vi "rszvl_core_global.vi"() -> ()   [LabVIEW 2014] (continued)
the settings of Bluetooth measurements.\n\n(2) Results (Class):\nAttributes that return the measured values and measurement results.", "Flags"={"OPC Wait"=FALSE, "Dont check status"=FALSE, "*WAI"=FALSE}, "Check Status Callback"=""}, {"Level"=2, "Descriptive Name"="Settings", "Class Only"=TRUE, "Data Type"=0, "Access"=0, "Identifier"="", "Range Table"="", "Command"="", "Read Callback"="", "Write Callback"="", "Range Callback"="", "Check Callback"="", "Rngtable Callback"="", "Coerce Callback"="", "User Callback"="", "Supported Models"="", "Instrument Options"="", "Repeated Capabilities"="", "Restricted Repeated Capabilities"="", "Help"="Attributes that configure the settings of Bluetooth measurements.\n\n(1) BTO Packet Type:\nThis attribute selects the packet type to be measured.\n\n(2) BTO Samples Per Symbols:\nThis attribute selects the number of measurement samples (points) per symbol for the measurement.\n\n(3) BTO Output Power Class:\nThis attribute selects the power class for the Output Power measurement. The power class defines the limits for the Output Power measurement.\n\n(4) BTO Position of Average Power:\nThis attribute defines the start/stop position for the calculation of the average power of a burst.\n\n(5) BTO Resolution Bandwidth Auto:\nThis attribute links the resolution bandwidth to the settings according to the RF Test Specification.\n\n(6) BTO Resolution Bandwidth:\nThis attribute sets the resolution bandwidth of the analyzer for the currently selected Bluetooth\nmeasurement\n\n(7) BTO Video Bandwidth Auto:\nThis attribute links the video bandwidth to the settings according to the RF Test Specification.\n\n(8) BTO Video Bandwidth:\nThis attribute sets the video bandwidth for the currently selected Bluetooth measurement.\n\n(9) BTO Measurement Filter:\nThis attribute selects the receive filter for the signal to measure.\n\n(10) BTO Trace Mode:\nThis attribute defines the way of displaying and evaluating the measurement curves for the\nselected Bluetooth measurement.\n\n(11) BTO Select Trace:\nThis attribute selects the measurement curve for evaluation of the modulation characteristics.\n\n(12) BTO Trace Detector:\nThis attribute selects the detector for the currently selected Bluetooth measurement. The numeric suffix assigns the detector to a trace.\n\n(13) BTO Sweep Count:\nThis attribute defines the number of sweeps for the currently selected Bluetooth measurement.\nThis number will be started as a single sweep.\n\n(14) BTO Sweep Time Auto:\nThis attribute links the sweep time to the settings according to the RF Test Specification.\n\n(15) BTO Sweep Time:\nThis attribute defines the duration of a sweep sequence for the active Bluetooth measurement.\n\n(16) BTO Mode:\nThis attribute selects the Bluetooth analyzer mode.\n\n(17) BTO Measurement Mode:\nThis attribute selects the current measurement according to the Bluetooth standard.\n\n(18) BTO Lowest 24 Bits of Bluetooth Device Address:\nThis attribute sets the lowest 24 bits of Bluetooth Device Address. These bits are used to determine the begin of the signal packet.\n\n(19) BTO Frequency Channel:\nThis attribute selects the frequency channel for the measurements according to the Bluetooth standard.\n\nNote:\nRange Tables rszvl_rngBtoChannel and rszvl_rngBtoChannelFranc are used for range checking.\n\n(20) BTO Number of Adjacent Channels:\nThis attribute selects the number of adjacent channel pairs during the measurement of the\nadjacent channel power. The number of adjacent channels will be limited as soon as the border of\nthe Bluetooth frequency band is reached.\n\n(21) BTO Geographical Region:\nThis attribute selects the geographical region for the measurements. The region determines the number of available frequency channels.\n\n(22) BTO Antenna Gain:\nThis attribute defines an external gain known to the analyzer, which will take it into account during\nthe display of measurement results. With this function the gain of an antenna or of an external\npreamplifier can be taken into account for the measurement values.\n\n(23) BTO Burst Offset:\nThis attribute defines the time to be recorded before a signal burst is recognized.\n\n(24) BTO Find Burst State:\nThis attribute switches the search for a signal burst on or off.\n\n(25) BTO Sync Offset:\nThis attribute defines the number of bits to be recorded before the first preamble bit is detected.\n\n(26) BTO Find Sync State:\nThis attribute switches the search for a sync pattern on or off.\n\n(27) BTO Search Time:\nThis attribute selects manual setting of the record length and defines the record length to be used\nfor the search of sync word and burst. The input of the record length is expected in seconds.\n\n(28) BTO Search Time Auto:\nThis attribute activates the automatic setting of the record length for the sync word and burst\nsearch, depending on the selected packet type.\n\n(29) BTO Carrier Frequency Stability Block Count:\nThis attribute sets the number of blocks to be measured.\n\nNote: \n\n(1) This command is only available with active Carrier Frequency Stability and Modulation Accuracy measurement\n\n(30) BTO Spurious Emissions Adjacent Channels:\nThis attribute selects the number of adjacent channel pairs during the In–band Spurious Emissions measurement. The number of adjacent channels will be limited as soon as the border of the Bluetooth frequency band is reached.\n\nNote: \n\n(1) This command is only available with active In–band Spurious Emissions measurement\n\n(31) BTO Spurious Emissions Gate Auto:\nThis attribute adjusts the gate settings for the In–band Spurious Emissions automatically.\n\nNote:\n\n(1) This command is only available with active In–band Spurious Emissions measurement\n\n(32) BTO Packet Bytes SCO:\nThis attribute selects the number of payload bytes that are transmitted in a packet.\n\n(33) BTO Relative Transimt Power Time:\nThis attribute sets the start/stop time for the power measurement of the DPSK or GFSK sections of the packet.\n\nNote: \n\n(1) This command is only available with active Relative Transmit Power measurement\n\n(34) BTO Y axis Scaling:\nThis attribute defines the scaling of the y–axis in the currently selected unit.\n\n(35) BTO Zoom:\nThis attribute enables or disables the zoom function.\n\nNote: \n\n(1) The zoom function is only available for the Output Power, Modulation Characteristics, Initial Carrier Frequency Tolerance, and Carrier Frequency Drift measurements.\n\n(36) BTO Zoom Start:\nThis attribute sets the start time for the display of individual measured values.\n\nNote: \n\n(1) The zoom function is only available for the Output Power, Modulation Characteristics, Initial Carrier Frequency Tolerance, and Carrier Frequency Drift measurements.", "Flags"={"OPC Wait"=FALSE, "Dont check status"=FALSE, "*WAI"=FALSE}, "Check Status Callback"=""}, {"Level"=3, "Descriptive Name"="BTO Packet Type", "Class Only"=FALSE, "Data Type"=0, "Access"=2, "Identifier"="RSZVL_ATTR_BTO_PTYPE", "Range Table"="rszvl_rngBtoWritePtype", "Command"="CONF:BTO:PTYP", "Read Callback"="", "Write Callback"="", "Range Callback"="", "Check Callback"="", "Rngtable Callback"="", "Coerce Callback"="", "User Callback"="", "Supported Models"="", "Instrument Options"="", "Repeated Capabilities"="", "Restricted Repeated Capabilities"="", "Help"="This attribute selects the packet type to be measured.\n\nAvailable Repeated Capabilities:\nNone\n\nRemote-control command(s):\nCONFigure:BTOoth:PTYPe DH1 | DH3 | DH5 | AUTO", "Flags"={"OPC Wait"=FALSE, "Dont check status"=FALSE, "*WAI"=FALSE}, "Check Status Callback"=""}, {"Level"=3, "Descriptive Name"="BTO Samples Per Symbols", "Class Only"=FALSE, "Data Type"=0, "Access"=2, "Identifier"="RSZVL_ATTR_BTO_PRAT", "Range Table"="rszvl_rngBtoPrat", "Command"="CONF:BTO:PRAT", "Read Callback"="", "Write Callback"="", "Range Callback"="", "Check Callback"="", "Rngtable Callback"="", "Coerce Callback"="", "User Callback"="", "Supported Models"="", "Instrument Options"="", "Repeated Capabilities"="", "Restricted Repeated Capabilities"="", "Help"="This attribute selects the number of measurement samples (points) per symbol for the measurement.\n\nAvailable Repeated Capabilities:\nNone\n\nRemote-control command(s):\nCONFigure:BTOoth:PRATe", "Flags"={"OPC Wait"=FALSE, "Dont check status"=FALSE, "*WAI"=FALSE}, "Check Status Callback"=""}, {"Level"=3, "Descriptive Name"="BTO Output Power Class", "Class Only"=FALSE, "Data Type"=0, "Access"=2, "Identifier"="RSZVL_ATTR_BTO_PCL", "Range Table"="rszvl_rngBtoPcl", "Command"="CONF:BTO:PCL", "Read Callback"="", "Write Callback"="", "Range Callback"="", "Check Callback"="", "Rngtable Callback"="", "Coerce Callback"="", "User Callback"="", "Supported Models"="", "Instrument Options"="", "Repeated Capabilities"="", "Restricted Repeated Capabilities"="", "Help"="This attribute selects the power class for the Output Power measurement. The power class defines the limits for the Output Power measurement.\n\nAvailable Repeated Capabilities:\nNone\n\nRemote-control command(s):\nCONFigure:BTOoth:PCLass", "Flags"={"OPC Wait"=FALSE, "Dont check status"=FALSE, "*WAI"=FALSE}, "Check Status Callback"=""}, {"Level"=3, "Descriptive Name"="BTO Position of Average Power", "Class Only"=FALSE, "Data Type"=1, "Access"=2, "Identifier"="RSZVL_ATTR_BTO_POW_AVER", "Range Table"="rszvl_rngPct", "Command"="CONF:BTO:POW:AVER:{ModifStopStart}", "Read Callback"="", "Write Callback"="", "Range Callback"="", "Check Callback"="", "Rngtable Callback"="", "Coerce Callback"="", "User Callback"="", "Supported Models"="", "Instrument Options"="", "Repeated Capabilities"="", "Restricted Repeated Capabilities"="", "Help"="This attribute defines the start/stop position for the calculation of the average power of a burst.\n\nAvailable Repeated Capabilities:\nModifStopStart: Stop,Start\r\n\nRemote-control command(s):\nCONFigure:BTOoth:POWer:AVERage:STARt|STOP", "Flags"={"OPC Wait"=FALSE, "Dont check status"=FALSE, "*WAI"=FALSE}, "Check Status Callback"=""}, {"Level"=3, "Descriptive Name"="BTO Resolution Bandwidth Auto", "Class Only"=FALSE, "Data Type"=3, "Access"=2, "Identifier"="RSZVL_ATTR_BTO_BWID_AUTO", "Range Table"="", "Command"="CONF:BTO:BWID:AUTO", "Read Callback"="", "Write Callback"="", "Range Callback"="", "Check Callback"="", "Rngtable Callback"="", "Coerce Callback"="", "User Callback"="", "Supported Models"="", "Instrument Options"="", "Repeated Capabilities"="", "Restricted Repeated Capabilities"="", "Help"="This attribute links the resolution bandwidth to the settings according to the RF Test Specification.\n\nAvailable Repeated Capabilities:\nNone\n\nRemote-control command(s):\nCONFigure:BTOoth:BANDwidth|BWIDth[:RESolution]:AUTO ON | OFF", "Flags"={"OPC Wait"=TRUE, "Dont check status"=FALSE, "*WAI"=FALSE}, "Check Status Callback"=""}, {"Level"=3, "Descriptive Name"="BTO Resolution Bandwidth", "Class Only"=FALSE, "Data Type"=1, "Access"=2, "Identifier"="RSZVL_ATTR_BTO_BWID", "Range Table"="rszvl_rngBtoBwid", "Command"="CONF:BTO:BWID:RES", "Read Callback"="", "Write Callback"="", "Range Callback"="", "Check Callback"="", "Rngtable Callback"="", "Coerce Callback"="", "User Callback"="", "Supported Models"="", "Instrument Options"="", "Repeated Capabilities"="", "Restricted Repeated Capabilities"="", "Help"="This attribute sets the resolution bandwidth of the analyzer for the currently selected Bluetooth\nmeasurement\n\nAvailable Repeated Capabilities:\nNone\n\nRemote-control command(s):\nCONFigure:BTOoth:BANDwidth|BWIDth[:RESolution]", "Flags"={"OPC Wait"=FALSE, "Dont check status"=FALSE, "*WAI"=FALSE}, "Check Status Callback"=""}, {"Level"=3, "Descriptive Name"="BTO Video Bandwidth Auto", "Class Only"=FALSE, "Data Type"=3, "Access"=2, "Identifier"="RSZVL_ATTR_BTO_VID_AUTO", "Range Table"="", "Command"="CONF:BTO:BWID:VID:AUTO", "Read Callback"="", "Write Callback"="", "Range Callback"="", "Check Callback"="", "Rngtable Callback"="", "Coerce Callback"="", "User Callback"="", "Supported Models"="", "Instrument Options"="", "Repeated Capabilities"="", "Restricted Repeated Capabilities"="", "Help"="This attribute links the video bandwidth to the settings according to the RF Test Specification.\n\nAvailable Repeated Capabilities:\nNone\n\nRemote-control command(s):\nCONFigure:BTOoth:BANDwidth|BWIDth:VIDeo:AUTO ON | OFF", "Flags"={"OPC Wait"=TRUE, "Dont check status"=FALSE, "*WAI"=FALSE}, "Check Status Callback"=""}, {"Level"=3, "Descriptive Name"="BTO Video Bandwidth", "Class Only"=FALSE, "Data Type"=1, "Access"=2, "Identifier"="RSZVL_ATTR_BTO_VID", "Range Table"="rszvl_rngBtoVideo", "Command"="CONF:BTO:BWID:VID", "Read Callback"="", "Write Callback"="", "Range Callback"="", "Check Callback"="", "Rngtable Callback"="", "Coerce Callback"="", "User Callback"="", "Supported Models"="", "Instrument Options"="", "Repeated Capabilities"="", "Restricted Repeated Capabilities"="", "Help"="This attribute sets the video bandwidth for the currently selected Bluetooth measurement.\n\nAvailable Repeated Capabilities:\nNone\n\nRemote-control command(s):\nCONFigure:BTOoth:BANDwidth|BWIDth:VIDeo", "Flags"={"OPC Wait"=FALSE, "Dont check status"=FALSE, "*WAI"=FALSE}, "Check Status Callback"=""}, {"Level"=3, "Descriptive Name"="BTO Measurement Filter", "Class Only"=FALSE, "Data Type"=0, "Access"=2, "Identifier"="RSZVL_ATTR_BTO_FILT_MEAS", "Range Table"="rszvl_rngBtoMeasFilt", "Command"="DDEM:FILT:MEAS", "Read Callback"="", "Write Callback"="", "Range Callback"="", "Check Callback"="", "Rngtable Callback"="", "Coerce Callback"="", "User Callback"="", "Supported Models"="", "Instrument Options"="", "Repeated Capabilities"="", "Restricted Repeated Capabilities"="", "Help"="This attribute selects the receive filter for the signal to measure.\n\nAvailable Repeated Capabilities:\nNone\n\nRemote-control command(s):\n[SENSe<1|2>:]DDEMod:FILTer:MEASurement OFF | BTOoth", "Flags"={"OPC Wait"=FALSE, "Dont check status"=FALSE, "*WAI"=FALSE}, "Check Status Callback"=""}, {"Level"=3, "Descriptive Name"="BTO Trace Mode", "Class Only"=FALSE, "Data Type"=0, "Access"=2, "Identifier"="RSZVL_ATTR_BTO_TRAC_MOD", "Range Table"="rszvl_rngTraceModeWithBlank", "Command"="CONF:BTO:TRAC{Trace}:MODE", "Read Callback"="", "Write Callback"="", "Range Callback"="", "Check Callback"="", "Rngtable Callback"="", "Coerce Callback"="", "User Callback"="", "Supported Models"="", "Instrument Options"="", "Repeated Capabilities"="", "Restricted Repeated Capabilities"="", "Help"="This attribute defines the way of displaying and evaluating the measurement curves for the selected Bluetooth measurement.\n\nAvailable Repeated Capabilities:\nTrace: TR1,TR2,TR3,TR4,TR5,TR6,TR7,TR8,TR9,TR10,TR11,TR12,TR13,TR14,TR15,TR16,TR17,TR18,TR19,TR20\r\n\nRemote-control command(s):\nCONFigure:BTOoth:TRACe<1...3>:MODE WRITe | VIEW | AVERage | BLANk | MAXHold | MINHold", "Flags"={"OPC Wait"=FALSE, "Dont check status"=FALSE, "*WAI"=FALSE}, "Check Status Callback"=""}, {"Level"=3, "Descriptive Name"="BTO Select Trace", "Class Only"=FALSE, "Data Type"=4, "Access"=1, "Identifier"="RSZVL_ATTR_BTO_TRAC", "Range Table"="", "Command"="CONF:BTO:TRAC{Trace}:SEL", "Read Callback"="", "Write Callback"="", "Range Callback"="", "Check Callback"="", "Rngtable Callback"="", "Coerce Callback"="", "User Callback"="", "Supported Models"="", "Instrument Options"="", "Repeated Capabilities"="", "Restricted Repeated Capabilities"="", "Help"="This attribute selects the measurement curve for evaluation of the modulation characteristics.\n\nAvailable Repeated Capabilities:\nTrace: TR1,TR2,TR3,TR4,TR5,TR6,TR7,TR8,TR9,TR10,TR11,TR12,TR13,TR14,TR15,TR16,TR17,TR18,TR19,TR20\r\n\nRemote-control command(s):\nCONFigure:BTOoth:TRACe<1...6>:SELect", "Flags"={"OPC Wait"=FALSE, "Dont check status"=FALSE, "*WAI"=FALSE}, "Check Status Callback"=""}, {"Level"=3, "Descriptive Name"="BTO Trace Detector", "Class Only"=FALSE, "Data Type"=0, "Access"=2, "Identifier"="RSZVL_ATTR_BTO_TRAC_DET", "Range Table"="rszvl_rngBtoTraceDetector", "Command"="CONF:BTO:DET{Trace}", "Read Callback"="", "Write Callback"="", "Range Callback"="", "Check Callback"="", "Rngtable Callback"="", "Coerce Callback"="", "User Callback"="", "Supported Models"="", "Instrument Options"="", "Repeated Capabilities"="", "Restricted Repeated Capabilities"="", "Help"="This attribute selects the detector for the currently selected Bluetooth measurement. The numeric suffix assigns the detector to a trace.\n\nAvailable Repeated Capabilities:\nTrace: TR1,TR2,TR3,TR4,TR5,TR6,TR7,TR8,TR9,TR10,TR11,TR12,TR13,TR14,TR15,TR16,TR17,TR18,TR19,TR20\r\n\nRemote-control command(s):\nCONFigure:BTOoth:DETector<1...4> APEak | NEGative | POSitive |SAMPle | RMS | AVERage", "Flags"={"OPC Wait"=FALSE, "Dont check status"=FALSE, "*WAI"=FALSE}, "Check Status Callback"=""}, {"Level"=3, "Descriptive Name"="BTO Sweep Count", "Class Only"=FALSE, "Data Type"=0, "Access"=2, "Identifier"="RSZVL_ATTR_BTO_SWE", "Range Table"="rszvl_rngSweepCount", "Command"="CONF:BTO:SWE:COUN", "Read Callback"="", "Write Callback"="", "Range Callback"="", "Check Callback"="", "Rngtable Callback"="", "Coerce Callback"="", "User Callback"="", "Supported Models"="", "Instrument Options"="", "Repeated Capabilities"="", "Restricted Repeated Capabilities"="", "Help"="This attribute defines the number of sweeps for the currently selected Bluetooth measurement.\nThis number will be started as a single sweep.\n\nAvailable Repeated Capabilities:\nNone\n\nRemote-control command(s):\nCONFigure:BTOoth:SWEep:COUNt", "Flags"={"OPC Wait"=FALSE, "Dont check status"=FALSE, "*WAI"=FALSE}, "Check Status Callback"=""}, {"Level"=3, "Descriptive Name"="BTO Sweep Time Auto", "Class Only"=FALSE, "Data Type"=3, "Access"=2, "Identifier"="RSZVL_ATTR_BTO_SWE_TIME_AUTO", "Range Table"="", "Command"="CONF:BTO:SWE:TIME:AUTO", "Read Callback"="", "Write Callback"="", "Range Callback"="", "Check Callback"="", "Rngtable Callback"="", "Coerce Callback"="", "User Callback"="", "Supported Models"="", "Instrument Options"="", "Repeated Capabilities"="", "Restricted Repeated Capabilities"="", "Help"="This attribute links the sweep time to the settings according to the RF Test Specification.\n\nAvailable Repeated Capabilities:\nNone\n\nRemote-control command(s):\nCONFigure:BTOoth:SWEep:TIME:AUTO ON | OFF", "Flags"={"OPC Wait"=TRUE, "Dont check status"=FALSE, "*WAI"=FALSE}, "Check Status Callback"=""}, {"Level"=3, "Descriptive Name"="BTO Sweep Time", "Class Only"=FALSE, "Data Type"=1, "Access"=2, "Identifier"="RSZVL_ATTR_BTO_SWE_TIME", "Range Table"="", "Command"="CONF:BTO:SWE:TIME", "Read Callback"="", "Write Callback"="", "Range Callback"="", "Check Callback"="", "Rngtable Callback"="", "Coerce Callback"="", "User Callback"="", "Supported Models"="", "Instrument Options"="", "Repeated Capabilities"="", "Restricted Repeated Capabilities"="", "Help"="This attribute defines the duration of a sweep sequence for the active Bluetooth measurement.\n\nAvailable Repeated Capabilities:\nNone\n\nRemote-control command(s):\nCONFigure:BTOoth:SWEep:TIME", "Flags"={"OPC Wait"=FALSE, "Dont check status"=FALSE, "*WAI"=FALSE}, "Check Status Callback"=""}, {"Level"=3, "Descriptive Name"="BTO Mode", "Class Only"=FALSE, "Data Type"=4, "Access"=1, "Identifier"="RSZVL_ATTR_BTO_MODE", "Range Table"="", "Command"="INST:SEL BTO", "Read Callback"="", "Write Callback"="", "Range Callback"="", "Check Callback"="", "Rngtable Callback"="", "Coerce Callback"="", "User Callback"="", "Supported Models"="", "Instrument Options"="", "Repeated Capabilities"="", "Restricted Repeated Capabilities"="", "Help"="This attribute selects the Bluetooth analyzer mode.\n\nAvailable Repeated Capabilities:\nNone\n\nRemote-control command(s):\nINSTrument<1|2>:SELect BTOoth", "Flags"={"OPC Wait"=FALSE, "Dont check status"=FALSE, "*WAI"=FALSE}, "Check Status Callback"=""}, {"Level"=3, "Descriptive Name"="BTO Measurement Mode", "Class Only"=FALSE, "Data Type"=0, "Access"=2, "Identifier"="RSZVL_ATTR_BTO", "Range Table"="rszvl_rngBtoMeasMode", "Command"="CONF:BTO:MEAS", "Read Callback"="", "Write Callback"="", "Range Callback"="", "Check Callback"="", "Rngtable Callback"="", "Coerce Callback"="", "User Callback"="", "Supported Models"="", "Instrument Options"="", "Repeated Capabilities"="", "Restricted Repeated Capabilities"="", "Help"="This attribute selects the current measurement according to the Bluetooth standard.\n\nAvailable Repeated Capabilities:\nNone\n\nRemote-control command(s):\nCONFigure:BTOoth:MEASurement OPOWer | ACLR | MCHar | ICFTolerance | CFDRift | RTPower | IBSemissions | DPENcoding | CFSTability", "Flags"={"OPC Wait"=FALSE, "Dont check status"=FALSE, "*WAI"=FALSE}, "Check Status Callback"=""}, {"Level"=3, "Descriptive Name"="BTO Lowest 24 Bits of Bluetooth Device Address", "Class Only"=FALSE, "Data Type"=0, "Access"=2, "Identifier"="RSZVL_ATTR_BTO_LAP", "Range Table"="", "Command"="SENS1:DDEM:SEAR:SYNC:LAP", "Read Callback"="rszvl_hex_ReadCallback.vi", "Write Callback"="rszvl_hex_WriteCallback.vi", "Range Callback"="", "Check Callback"="", "Rngtable Callback"="", "Coerce Callback"="", "User Callback"="", "Supported Models"="", "Instrument Options"="", "Repeated Capabilities"="", "Restricted Repeated Capabilities"="", "Help"="This attribute sets the lowest 24 bits of Bluetooth Device Address. These bits are used to determine the begin of the signal packet.\n\nAvailable Repeated Capabilities:\nNone\n\nRemote-control command(s):\n[SENSe<1|2>:]DDEMod:SEARch:SYNC:LAP", "Flags"={"OPC Wait"=FALSE, "Dont check status"=FALSE, "*WAI"=FALSE}, "Check Status Callback"=""}, {"Level"=3, "Descriptive Name"="BTO Frequency Channel", "Class Only"=FALSE, "Data Type"=0, "Access"=2, "Identifier"="RSZVL_ATTR_BTO_CHANNEL", "Range Table"="rszvl_rngBtoChannel", "Command"="CONF:BTO:CHAN", "Read Callback"="", "Write Callback"="", "Range Callback"="", "Check Callback"="", "Rngtable Callback"="", "Coerce Callback"="", "User Callback"="", "Supported Models"="", "Instrument Options"="", "Repeated Capabilities"="", "Restricted Repeated Capabilities"="", "Help"="This attribute selects the frequency channel for the measurements according to the Bluetooth standard.\n\nAvailable Repeated Capabilities:\nNone\n\nRemote-control command(s):\nCONFigure:BTOoth:CHANnel", "Flags"={"OPC Wait"=FALSE, "Dont check status"=FALSE, "*WAI"=FALSE}, "Check Status Callback"=""}, {"Level"=3, "Descriptive Name"="BTO Number of Adjacent Channels", "Class Only"=FALSE, "Data Type"=0, "Access"=2, "Identifier"="RSZVL_ATTR_BTO_ACLR_ACP", "Range Table"="rszvl_rngBtoAclrAcp", "Command"="CONF:BTO:ACLR:ACP", "Read Callback"="", "Write Callback"="", "Range Callback"="", "Check Callback"="", "Rngtable Callback"="", "Coerce Callback"="", "User Callback"="", "Supported Models"="", "Instrument Options"="", "Repeated Capabilities"="", "Restricted Repeated Capabilities"="", "Help"="This attribute selects the number of adjacent channel pairs during the measurement of the\nadjacent channel power. The number of adjacent channels will be limited as soon as the border of\nthe Bluetooth frequency band is reached.\n\nAvailable Repeated Capabilities:\nNone\n\nRemote-control command(s):\nCONFigure:BTOoth:ACLR:ACPairs", "Flags"={"OPC Wait"=FALSE, "Dont check status"=FALSE, "*WAI"=FALSE}, "Check Status Callback"=""}, {"Level"=3, "Descriptive Name"="BTO Antenna Gain", "Class Only"=FALSE, "Data Type"=1, "Access"=2, "Identifier"="RSZVL_ATTR_BTO_EGA_INP", "Range Table"="rszvl_rngBtoAntennaGain", "Command"="CORR:EGA:INP", "Read Callback"="", "Write Callback"="", "Range Callback"="", "Check Callback"="", "Rngtable Callback"="", "Coerce Callback"="", "User Callback"="", "Supported Models"="", "Instrument Options"="", "Repeated Capabilities"="", "Restricted Repeated Capabilities"="", "Help"="This attribute defines an external gain known to the analyzer, which will take it into account during\nthe display of measurement results. With this function the gain of an antenna or of an external\npreamplifier can be taken into account for the measurement values.\n\nAvailable Repeated Capabilities:\nNone\n\nRemote-control command(s):\n[SENSe<1|2>:]CORRection:EGAin:INPut[:MAGNitude]", "Flags"={"OPC Wait"=FALSE, "Dont check status"=FALSE, "*WAI"=FALSE}, "Check Status Callback"=""}, {"Level"=3, "Descriptive Name"="BTO Burst Offset", "Class Only"=FALSE, "Data Type"=1, "Access"=2, "Identifier"="RSZVL_ATTR_BTO_PULS_OFFS", "Range Table"="rszvl_rngBtoBurstOffs", "Command"="DDEM:SEAR:PULS:OFFS", "Read Callback"="", "Write Callback"="", "Range Callback"="", "Check Callback"="", "Rngtable Callback"="", "Coerce Callback"="", "User Callback"="", "Supported Models"="", "Instrument Options"="", "Repeated Capabilities"="", "Restricted Repeated Capabilities"="", "Help"="This attribute defines the time to be recorded before a signal burst is recognized.\n\nAvailable Repeated Capabilities:\nNone\n\nRemote-control command(s):\n[SENSe<1|2>:]DDEMod:SEARch:PULSe:OFFSet", "Flags"={"OPC Wait"=FALSE, "Dont check status"=FALSE, "*WAI"=FALSE}, "Check Status Callback"=""}, {"Level"=3, "Descriptive Name"="BTO Find Burst State", "Class Only"=FALSE, "Data Type"=3, "Access"=2, "Identifier"="RSZVL_ATTR_BTO_SEARCH_PULS", "Range Table"="", "Command"="DDEM:SEAR:PULS", "Read Callback"="", "Write Callback"="", "Range Callback"="", "Check Callback"="", "Rngtable Callback"="", "Coerce Callback"="", "User Callback"="", "Supported Models"="", "Instrument Options"="", "Repeated Capabilities"="", "Restricted Repeated Capabilities"="", "Help"="This attribute switches the search for a signal burst on or off.\n\nAvailable Repeated Capabilities:\nNone\n\nRemote-control command(s):\n[SENSe<1|2>:]DDEMod:SEARch:PULSe[:STATe] ON | OFF", "Flags"={"OPC Wait"=FALSE, "Dont check status"=FALSE, "*WAI"=FALSE}, "Check Status Callback"=""}, {"Level"=3, "Descriptive Name"="BTO Sync Offset", "Class Only"=FALSE, "Data Type"=0, "Access"=2, "Identifier"="RSZVL_ATTR_BTO_SYNC_OFFS", "Range Table"="rszvl_rngBtoSyncOffs", "Command"="DDEM:SEAR:SYNC:OFFS", "Read Callback"="", "Write Callback"="", "Range Callback"="", "Check Callback"="", "Rngtable Callback"="", "Coerce Callback"="", "User Callback"="", "Supported Models"="", "Instrument Options"="", "Repeated Capabilities"="", "Restricted Repeated Capabilities"="", "Help"="This attribute defines the number of bits to be recorded before the first preamble bit is detected.\n\nAvailable Repeated Capabilities:\nNone\n\nRemote-control command(s):\n[SENSe<1|2>:]DDEMod:SEARch:SYNC:OFFSet", "Flags"={"OPC Wait"=FALSE, "Dont check status"=FALSE, "*WAI"=FALSE}, "Check Status Callback"=""}, {"Level"=3, "Descriptive Name"="BTO Find Sync State", "Class Only"=FALSE, "Data Type"=3, "Access"=2, "Identifier"="RSZVL_ATTR_BTO_SEARCH_SYNC", "Range Table"="", "Command"="DDEM:SEAR:SYNC", "Read Callback"="", "Write Callback"="", "Range Callback"="", "Check Callback"="", "Rngtable Callback"="", "Coerce Callback"="", "User Callback"="", "Supported Models"="", "Instrument Options"="", "Repeated Capabilities"="", "Restricted Repeated Capabilities"="", "Help"="This attribute switches the search for a sync pattern on or off.\n\nAvailable Repeated Capabilities:\nNone\n\nRemote-control command(s):\n[SENSe<1|2>:]DDEMod:SEARch:SYNC[:STATe]", "Flags"={"OPC Wait"=FALSE, "Dont check status"=FALSE, "*WAI"=FALSE}, "Check Status Callback"=""}, {"Level"=3, "Descriptive Name"="BTO Search Time", "Class Only"=FALSE, "Data Type"=1, "Access"=2, "Identifier"="RSZVL_ATTR_BTO_SEARCH_TIME", "Range Table"="rszvl_rngBtoSearchTime", "Command"="DDEM:SEAR:TIME", "Read Callback"="", "Write Callback"="", "Range Callback"="", "Check Callback"="", "Rngtable Callback"="", "Coerce Callback"="", "User Callback"="", "Supported Models"="", "Instrument Options"="", "Repeated Capabilities"="", "Restricted Repeated Capabilities"="", "Help"="This attribute selects manual setting of the record length and defines the record length to be used\nfor the search of sync word and burst. The input of the record length is expected in seconds.\n\nAvailable Repeated Capabilities:\nNone\n\nRemote-control command(s):\n[SENSe<1|2>:]DDEMod:SEARch:TIME", "Flags"={"OPC Wait"=FALSE, "Dont check status"=FALSE, "*WAI"=FALSE}, "Check Status Callback"=""}, {"Level"=3, "Descriptive Name"="BTO Search Time Auto", "Class Only"=FALSE, "Data Type"=3, "Access"=2, "Identifier"="RSZVL_ATTR_BTO_SEARCH_TIME_AUTO", "Range Table"="", "Command"="DDEM:SEAR:TIME:AUTO", "Read Callback"="", "Write Callback"="", "Range Callback"="", "Check Callback"="", "Rngtable Callback"="", "Coerce Callback"="", "User Callback"="", "Supported Models"="", "Instrument Options"="", "Repeated Capabilities"="", "Restricted Repeated Capabilities"="", "Help"="This attribute activates the automatic setting of the record length for the sync word and burst\nsearch, depending on the selected packet type.\n\nAvailable Repeated Capabilities:\nNone\n\nRemote-control command(s):\n[SENSe<1|2>:]DDEMod:SEARch:TIME:AUTO ON | OFF", "Flags"={"OPC Wait"=FALSE, "Dont check status"=FALSE, "*WAI"=FALSE}, "Check Status Callback"=""}, {"Level"=3, "Descriptive Name"="BTO Carrier Frequency Stability Block Count", "Class Only"=FALSE, "Data Type"=0, "Access"=2, "Identifier"="RSZVL_ATTR_BTO_CFST_BLOCK_COUNT", "Range Table"="rszvl_rngBtoCfstBlockCount", "Command"="CONF:BTO:CFST:BCO", "Read Callback"="", "Write Callback"="", "Range Callback"="", "Check Callback"="", "Rngtable Callback"="", "Coerce Callback"="", "User Callback"="", "Supported Models"="", "Instrument Options"="", "Repeated Capabilities"="", "Restricted Repeated Capabilities"="", "Help"="This attribute sets the number of blocks to be measured.\n\nNote: \n\n(1) This command is only available with active Carrier Frequency Stability and Modulation Accuracy measurement\n\nAvailable Repeated Capabilities:\nNone\n\nRemote-control command(s):\nCONFigure:BTOoth:CFSTability:BCOunt", "Flags"={"OPC Wait"=FALSE, "Dont check status"=FALSE, "*WAI"=FALSE}, "Check Status Callback"=""}, {"Level"=3, "Descriptive Name"="BTO Spurious Emissions Adjacent Channels", "Class Only"=FALSE, "Data Type"=0, "Access"=2, "Identifier"="RSZVL_ATTR_BTO_IBS_ACP", "Range Table"="rszvl_rngBtoAclrAcp", "Command"="CONF:BTO:IBS:ACP", "Read Callback"="", "Write Callback"="", "Range Callback"="", "Check Callback"="", "Rngtable Callback"="", "Coerce Callback"="", "User Callback"="", "Supported Models"="", "Instrument Options"="", "Repeated Capabilities"="", "Restricted Repeated Capabilities"="", "Help"="This attribute selects the number of adjacent channel pairs during the In–band Spurious Emissions measurement. The number of adjacent channels will be limited as soon as the border of the Bluetooth frequency band is reached.\n\nNote: \n\n(1) This command is only available with active In–band Spurious Emissions measurement\n\nAvailable Repeated Capabilities:\nNone\n\nRemote-control command(s):\nCONFigure:BTOoth:IBSemissions:ACPairs", "Flags"={"OPC Wait"=FALSE, "Dont check status"=FALSE, "*WAI"=FALSE}, "Check Status Callback"=""}, {"Level"=3, "Descriptive Name"="BTO Spurious Emissions Gate Auto", "Class Only"=FALSE, "Data Type"=4, "Access"=1, "Identifier"="RSZVL_ATTR_BTO_IBS_GATE_AUTO", "Range Table"="", "Command"="CONF:BTO:IBS:GATE:AUTO ONCE", "Read Callback"="", "Write Callback"="", "Range Callback"="", "Check Callback"="", "Rngtable Callback"="", "Coerce Callback"="", "User Callback"="", "Supported Models"="", "Instrument Options"="", "Repeated Capabilities"="", "Restricted Repeated Capabilities"="", "Help"="This attribute adjusts the gate settings for the In–band Spurious Emissions automatically.\n\nNote:\n\n(1) This command is only available with active In–band Spurious Emissions measurement\n\nAvailable Repeated Capabilities:\nNone\n\nRemote-control command(s):\nCONFigure:BTOoth:IBSemissions:GATE:AUTO ONCE", "Flags"={"OPC Wait"=FALSE, "Dont check status"=FALSE, "*WAI"=FALSE}, "Check Status Callback"=""}, {"Level"=3, "Descriptive Name"="BTO Packet Bytes SCO", "Class Only"=FALSE, "Data Type"=0, "Access"=2, "Identifier"="RSZVL_ATTR_BTO_PBSC", "Range Table"="rszvl_rngBtoPayloadBytes", "Command"="CONF:BTO:PBSC", "Read Callback"="", "Write Callback"="", "Range Callback"="", "Check Callback"="", "Rngtable Callback"="", "Coerce Callback"="", "User Callback"="", "Supported Models"="", "Instrument Options"="", "Repeated Capabilities"="", "Restricted Repeated Capabilities"="", "Help"="This attribute selects the number of payload bytes that are transmitted in a packet.\n\nAvailable Repeated Capabilities:\nNone\n\nRemote-control command(s):\nCONFigure:BTOoth:PBSCo", "Flags"={"OPC Wait"=FALSE, "Dont check status"=FALSE, "*WAI"=FALSE}, "Check Status Callback"=""}, {"Level"=3, "Descriptive Name"="BTO Relative Transimt Power Time", "Class Only"=FALSE, "Data Type"=1, "Access"=2, "Identifier"="RSZVL_ATTR_BTO_RTP_TIME", "Range Table"="rszvl_rngPct", "Command"="CONF:BTO:RTP:{BtoRtpTimePacketSection}:{ModifStopStart}", "Read Callback"="", "Write Callback"="", "Range Callback"="", "Check Callback"="", "Rngtable Callback"="", "Coerce Callback"="", "User Callback"="", "Supported Models"="", "Instrument Options"="", "Repeated Capabilities"="", "Restricted Repeated Capabilities"="", "Help"="This attribute sets the start/stop time for the power measurement of the DPSK or GFSK sections of the packet.\n\nNote: \n\n(1) This command is only available with active Relative Transmit Power measurement\n\nAvailable Repeated Capabilities:\nBtoRtpTimePacketSection: SECTION_TIME_GFSK,SECTION_TIME_DPSK\r\nModifStopStart: Stop,Start\r\n\nRemote-control command(s):\nCONFigure:BTOoth:RTPower:<DAVerage | :GAVerage>:STARt | STOP", "Flags"={"OPC Wait"=FALSE, "Dont check status"=FALSE, "*WAI"=FALSE}, "Check Status Callback"=""}, {"Level"=3, "Descriptive Name"="BTO Y axis Scaling", "Class Only"=FALSE, "Data Type"=1, "Access"=2, "Identifier"="RSZVL_ATTR_BTO_PDIV", "Range Table"="", "Command"="DISP:TRAC:Y:PDIV", "Read Callback"="", "Write Callback"="", "Range Callback"="", "Check Callback"="", "Rngtable Callback"="", "Coerce Callback"="", "User Callback"="", "Supported Models"="", "Instrument Options"="", "Repeated Capabilities"="", "Restricted Repeated Capabilities"="", "Help"="This attribute defines the scaling of the y–axis in the currently selected unit.\n\nAvailable Repeated Capabilities:\nNone\n\nRemote-control command(s):\nDISPlay[:WINDow<1|2>]:TRACE<1...6>:Y[:SCALe]:PDIVision", "Flags"={"OPC Wait"=FALSE, "Dont check status"=FALSE, "*WAI"=FALSE}, "Check Status Callback"=""}, {"Level"=3, "Descriptive Name"="BTO Zoom", "Class Only"=FALSE, "Data Type"=3, "Access"=2, "Identifier"="RSZVL_ATTR_BTO_ZOOM_STATE", "Range Table"="", "Command"="ADEM:ZOOM", "Read Callback"="", "Write Callback"="", "Range Callback"="", "Check Callback"="", "Rngtable Callback"="", "Coerce Callback"="", "User Callback"="", "Supported Models"="", "Instrument Options"="", "Repeated Capabilities"="", "Restricted Repeated Capabilities"="", "Help"="This attribute enables or disables the zoom function.\n\nNote: \n\n(1) The zoom function is only available for the Output Power, Modulation Characteristics, Initial Carrier Frequency Tolerance, and Carrier Frequency Drift measurements.\n\nAvailable Repeated Capabilities:\nNone\n\nRemote-control command(s):\n[SENSe:]ADEMod:ZOOM[:STATe]", "Flags"={"OPC Wait"=FALSE, "Dont check status"=FALSE, "*WAI"=FALSE}, "Check Status Callback"=""}, {"Level"=3, "Descriptive Name"="BTO Zoom Start", "Class Only"=FALSE, "Data Type"=1, "Access"=2, "Identifier"="RSZVL_ATTR_BTO_ZOOM_START", "Range Table"="", "Command"="ADEM:ZOOM:STAR", "Read Callback"="", "Write Callback"="", "Range Callback"="", "Check Callback"="", "Rngtable Callback"="", "Coerce Callback"="", "User Callback"="", "Supported Models"="", "Instrument Options"="", "Repeated Capabilities"="", "Restricted Repeated Capabilities"="", "Help"="This attribute sets the start time for the display of individual measured values.\n\nNote: \n\n(1) The zoom function is only available for the Output Power, Modulation Characteristics, Initial Carrier Frequency Tolerance, and Carrier Frequency Drift measurements.\n\nAvailable Repeated Capabilities:\nNone\n\nRemote-control command(s):\n[SENSe:]ADEMod:ZOOM:STARt", "Flags"={"OPC Wait"=FALSE, "Dont check status"=FALSE, "*WAI"=FALSE}, "Check Status Callback"=""}, {"Level"=2, "Descriptive Name"="Results", "Class Only"=TRUE, "Data Type"=0, "Access"=0, "Identifier"="", "Range Table"="", "Command"="", "Read Callback"="", "Write Callback"="", "Range Callback"="", "Check Callback"="", "Rngtable Callback"="", "Coerce Callback"="", "User Callback"="", "Supported Models"="", "Instrument Options"="", "Repeated Capabilities"="", "Restricted Repeated Capabilities"="", "Help"="Attributes that return the measured values and measurement results.\n\n(1) BTO Get Output Power Peak:\nThis attribute returns the peak value of the Output Power Measurement according to the BLUETOOTH standard.\n\n(2) BTO Get Output Power Average:\nThis attribute reads the average value of the Output Power measurement according to the Bluetooth standard.\n\n(3) BTO Get Status:\nThis attribute queries the status of a preceeding measurement.\n\n0: PASS\n1: FAIL\n\n(4) BTO Get Number Of Exceptions:\nThis attribute returns the number of exceptions which occured during the adjacent channel\npower measurement according to the Bluetooth specification.\n\n(5) BTO Get Average Frequency Deviation:\nThis attribute returns the value of average frequency deviation for varying bit patterns of the payload.\n\n(6) BTO Get Maximum Frequency Deviation Value:\nThis attribute returns the value of maximum frequency deviation for different bit patterns of the payload.\n\n(7) BTO Get Ratio Of Average Frequency Deviations Value:\nThis attribute returns the value of ratio of the average frequency deviations for varying bit patterns of the payload.\n\n(8) BTO Get Percentage Deviation:\nThis attribute returns the percentage of measurements of the frequency deviation.\n\n(9) BTO Get Initial Carrier Frequency Tolerance Value:\nThis attribute returns value of the Initial Carrier Frequency Tolerance.\n\nNote(s):\n(1) This command is only available with active Initial Carrier Frequency Tolerance measurement (command CONF:BTO:MEAS ICFT). With all other measurements this command will lead to a query error.\n\n(10) BTO Get Maximum Carrier Frequency Drift:\nThis attribute returns the maximum Carrier Frequency Drift.\n\nNote(s):\n(1) This command is only available with active Carrier Frequency Drift measurement (command CONF:BTO:MEAS CFDR). With all other measurements this command will lead to a query error.\n\n(11) BTO Get Carrier Frequency Drift:\nThis attribute returns the maximum Carrier Frequency Drift per 50 ms.\n\nNote(s):\n(1) This command is only available with active Carrier Frequency Drift measurement (command CONF:BTO:MEAS CFDR). With all other measurements this command will lead to a query error.\n\n(12) BTO Get Packet Length:\nThis attribute returns the length of the packet analyzed by the preceeding measurement.\n\n(13) BTO Get Packet Type:\nThis attribute returns the type of the packet analyzed by a preceeding measurement.\n\n(14) BTO Get Measured Block:\nThis attribute reads the number of measured blocks during or after a measurement.\n\nNote:\n\n(1) This command is only available with active Carrier Frequency Stability and Modulation\nAccuracy measurement.\n\n(15) BTO Get Modulation Accuracy of DEVM RMS :\nThis attribute reads the RMAS of differential error vector magnitude (DEVM) in the Carrier Frequency Stability and Modulation Accuracy measurement.\n\nNote:\n\n(1) This command is only available with active Carrier Frequency Stability and Modulation\nAccuracy measurement.\n\n(16) BTO Get Modulation Accuracy of DEVM Peak:\nThis attribute reads the Peak of differential error vector magnitude (DEVM) in the Carrier Frequency Stability and Modulation Accuracy measurement.\n\nNote:\n\n(1) This command is only available with active Carrier Frequency Stability and Modulation\nAccuracy measurement.\n\n(17)
